vi "selectAutonMode.vi"(2 "Auton File":dbl) -> ()   [LabVIEW 2011]
uses:
  <vilib>/Rock Robotics/WPI/DriverStation/DriverStationLCD/WPI_DriverStationLCDLCDLine.ctl
  Robot Global Data.vi
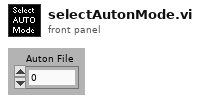
[diagram p1: front panel]
types:
  T1 = typedef "WPI_DriverStationLCDLCDLine.ctl" = enum16{"Main - Line 1", "User - Line 2", "User - Line 3", "User - Line 4", "User - Line 5", "User - Line 6"}
  T2 = enum16{"False", "FalseToTrue", "True", "TrueToFalse"}
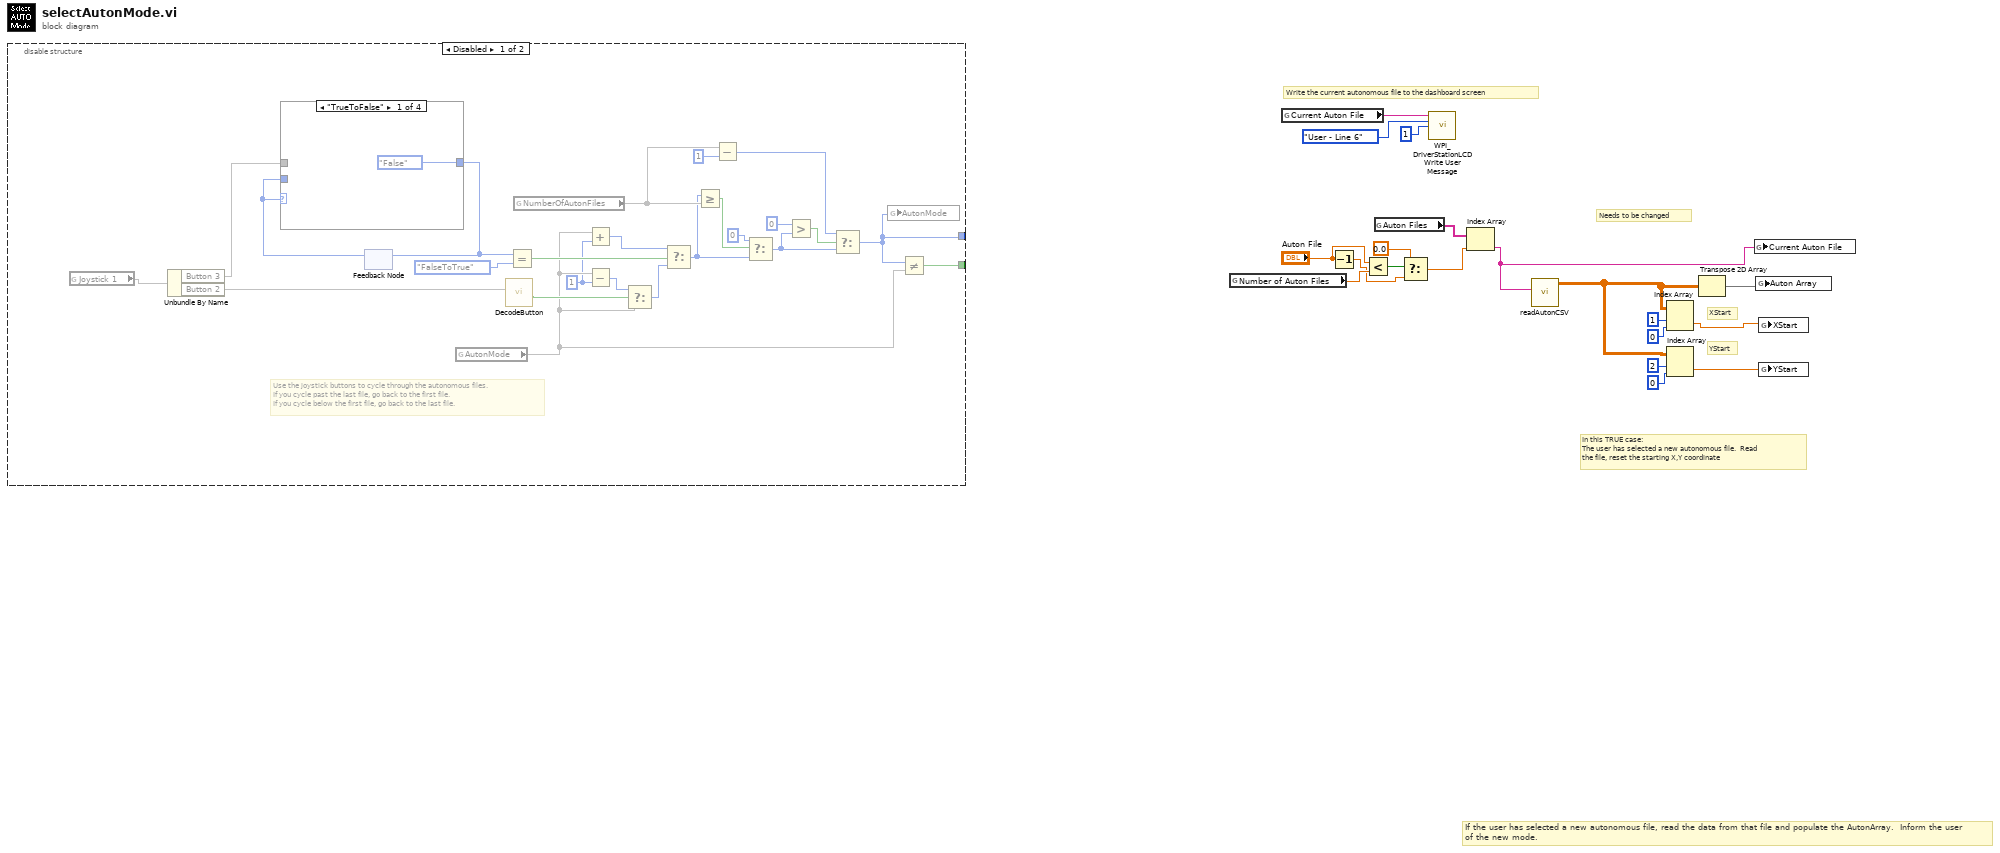
[diagram p0: block diagram]
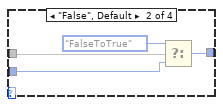
[diagram p2: hidden frame]
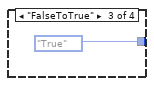
[diagram p3: hidden frame]
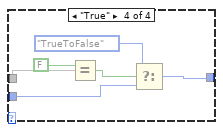
[diagram p4: hidden frame]
diagram:
  # "Needs to be changed"
  # "In this TRUE case:\nThe user has selected a new autonomous file.  Read\nthe file, reset the starting X,Y coordinate"
  # "YStart"
  # "XStart"
  # "Write the current autonomous file to the dashboard screen"
  # "If the user has selected a new autonomous file, read the data from that file and populate the AutonArray.  Inform the user\nof the new mode."
  n1 = disable-structure shown="Disabled" {
    disable-tunnel: [w43 _] -> _
    disable-tunnel: [w33 _] -> _
    frame Disabled {
      w24 = i16 1 ("y")
      # "Use the joystick buttons to cycle through the autonomous files.\nIf you cycle past the last file, go back to the first file.\nIf you cycle below the first file, go back to the last file."
      n2 = global read "Robot Global Data.vi" "Joystick 1"() -> (w20)
      n3 = Unbundle By Name(w20) -> ("Button 3"=w31, "Button 2"=w21)
      n4 = feedback #1() -> (w28:T2)  [unwired: 1 out]
      n5 = case shown="\"TrueToFalse\"" w28 {
        tunnel: w31 -> [_ w48 _ w54]
        tunnel: [T2."False" ("f") w46 T2."True" ("y") w55] -> w29
        tunnel: w28 -> [_ w45 _ w51]
        frame "TrueToFalse" {
        }
        frame "False", Default {
          n6 = Select(t=T2."FalseToTrue", s=w48, f=w45) -> (s? t:f=w46:T2)
        }
        frame "FalseToTrue" {
        }
        frame "True" {
          n7 = Equal?(x=FALSE, y=w54) -> (x = y?=w52:bool)
          n8 = Select(t=T2."TrueToFalse", s=w52, f=w51) -> (s? t:f=w55:T2)
        }
      }
      n9 = feedback-in #1(w29) -> ()
      n10 = global read "Robot Global Data.vi" "AutonMode"() -> (w26)
      n11 = call "DecodeButton.vi"("Button"=w21) -> ("False to True"=w27:bool)  [unwired: 10 out]
      n12 = Equal?(x=w29, y=T2."FalseToTrue") -> (x = y?=w32:bool)
      n13 = global read "Robot Global Data.vi" "NumberOfAutonFiles"() -> (w40)
      n14 = Add(x=w26, y=w24) -> (x+y=w25:i16)
      n15 = Subtract(x=w26, y=w24) -> (x-y=w22:i16)
      n16 = Select(t=w22, s=w27, f=w26) -> (s? t:f=w23:i16)
      n17 = Select(t=w25, s=w32, f=w23) -> (s? t:f=w34:i16)
      n18 = Greater Or Equal?(x=w34, y=w40) -> (x >= y?=w35:bool)
      n19 = Subtract(x=w40, y=i16 1) -> (x-y=w42:i16)
      n20 = Select(t=i16 0, s=w35, f=w34) -> (s? t:f=w37:i16)
      n21 = Greater?(x=i16 0, y=w37) -> (0:w39:bool)
      n22 = Select(t=w42, s=w39, f=w37) -> (s? t:f=w43:i16)
      n23 = global write "Robot Global Data.vi" "AutonMode"(w43) -> ()
      n24 = Not Equal?(x=w43, y=w26) -> (x != y?=w33:bool)
    }
    frame Enabled {
    }
  }
  n25 = global read "Robot Global Data.vi" "Number of Auton Files"() -> (w6:dbl)
  n26 = global read "Robot Global Data.vi" "Current Auton File"() -> (w13:string)
  n27 = Decrement(x="Auton File") -> (x-1=w1:dbl)
  n28 = Less?(x="Auton File", y=w6) -> (x < y?=w5:bool)
  n29 = global read "Robot Global Data.vi" "Auton Files"() -> (w12:string[])
  n30 = Select(t=0.0, s=w5, f=w1) -> (s? t:f=w3:dbl)
  n31 = call <vilib>:"WPI_DriverStationLCDWrite User Message.vi"("line text"=w13, "line"=WPI_DriverStationLCDLCDLine."User - Line 6", "starting column"=i8 1) -> ()  [unwired: 2 in, 11 out]
  n32 = Index Array(array=w12, index=w3) -> (element=w9:string)
  n33 = call "readAutonCSV.vi"("AutonFile"=w9) -> ("AutonArray"=w8:dbl[][])  [unwired: 7 out]
  n34 = Index Array(array=w8, index (row)=1 ("disabled index (row)"), index (col)=0) -> (element=w11:dbl)
  n35 = Index Array(array=w8, index (row)=2 ("disabled index (row)"), index (col)=0) -> (element=w10:dbl)
  n36 = Transpose 2D Array(2D array=w8) -> (transposed array=w7:dbl[][])
  n37 = global write "Robot Global Data.vi" "Current Auton File"(w9) -> ()
  n38 = global write "Robot Global Data.vi" "Auton Array"(w7) -> ()
  n39 = global write "Robot Global Data.vi" "XStart"(w11) -> ()
  n40 = global write "Robot Global Data.vi" "YStart"(w10) -> ()
